vi "addAmountToStringArray.vi"(8 "error in (no error)":errorcluster, 10 "Array In":string[](array[string]), 11 "UserEditableAmount in":refnum<class "UserEditableAmount.lvclass">) -> (0 "error out":errorcluster, 2 "Array Out":string[](array[string]), 3 "UserEditableAmount out":refnum<class "UserEditableAmount.lvclass">)   [LabVIEW 2018, in "UserEditableAmount.lvclass"]
uses:
  UserEditableAmount.lvclass
  UserEditableAmount.lvclass/UserEditableAmount.ctl
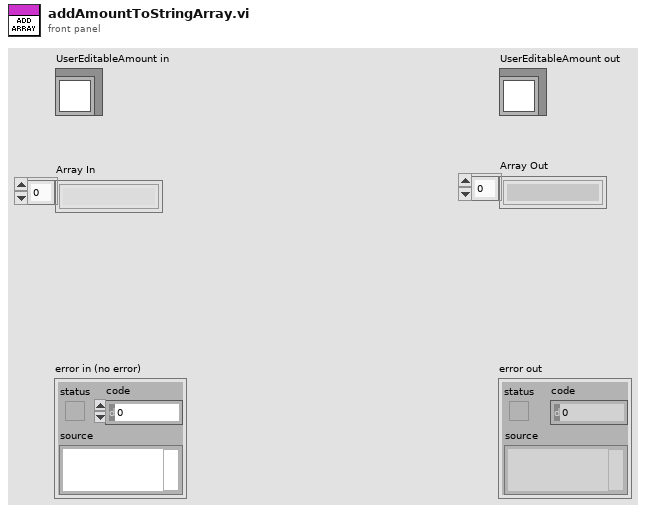
[diagram p1: front panel]
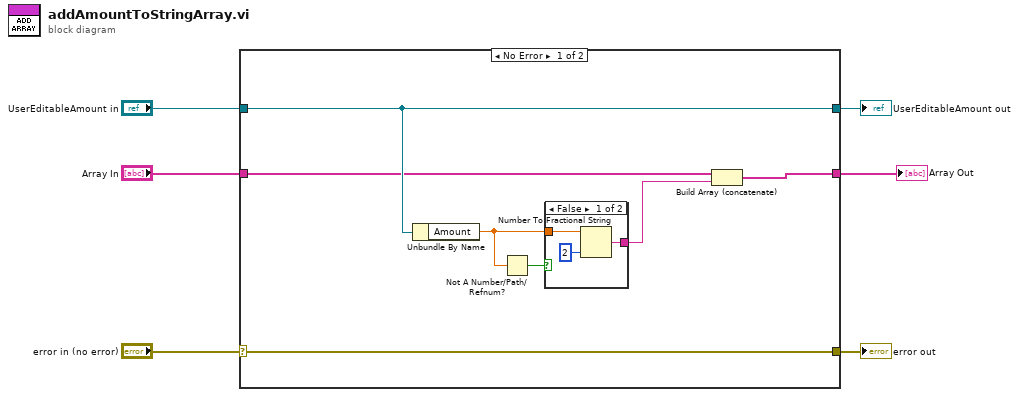
[diagram p0: block diagram]
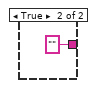
[diagram p2: hidden frame]
diagram:
  n1 = case shown="No Error" "error in (no error)" {
    selector: "error in (no error)" -> [w13 w20]
    tunnel: [w13 w20] -> w5
    tunnel: [w11 w19] -> w3
    tunnel: "UserEditableAmount in" -> [w11 w19]
    tunnel: "Array In" -> [w9 w18]
    tunnel: [w7 w18] -> w1
    frame No Error {
      n2 = Unbundle By Name(w11) -> ("Amount"=w10:dbl)
      n3 = Not A Number/Path/Refnum?(number/path/refnum=w10) -> (NaN/Path/Refnum?=w12:bool)
      n4 = case shown="False" w12 {
        tunnel: [w15 ""] -> w8
        tunnel: w10 -> [w14 _]
        frame False {
          n5 = Number To Fractional String(number=w14, precision (6)=i16 2) -> (F-format string=w15:string)  [unwired: 2 in]
        }
        frame True {
        }
      }
      n6 = Build Array (concatenate)(w9, w8) -> (w7:string[])
    }
    frame Error {
    }
  }
  "error out" <- w5
  "UserEditableAmount out" <- w3
  "Array Out" <- w1
